vi "Convert RGB 1D Array to U32.vi"(9 "height":i32, 10 "width":i32, 11 "image":u8[](array[numeric])) -> (3 "output array":u32[][](array[numeric]) format="%.0x")   [LabVIEW 2025]
panel:
  out "?":u64[](array[numeric]) format="%.0x"
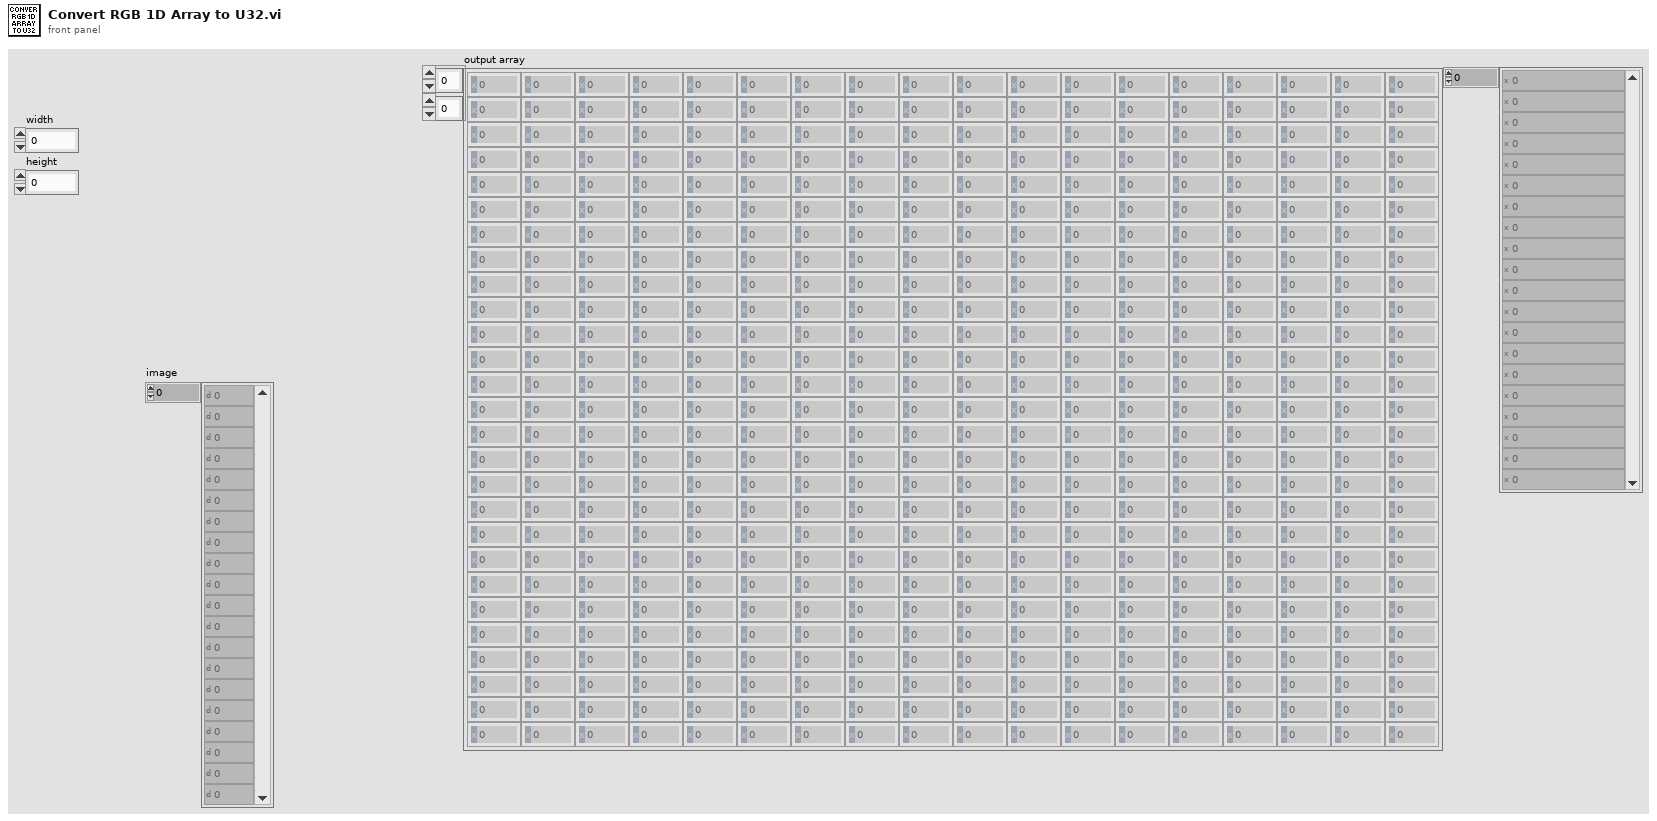
[diagram p1: front panel]
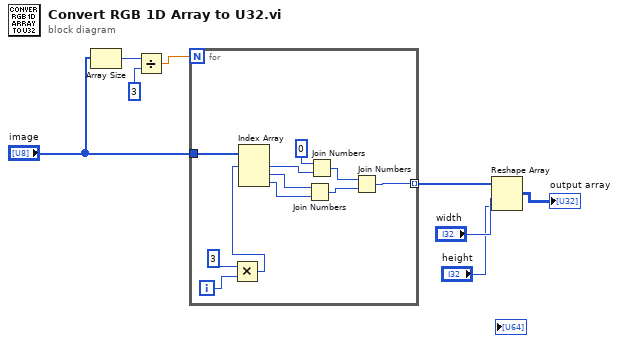
[diagram p0: block diagram]
diagram:
  n1 = Array Size(array="image") -> (size(s)=w4:i32)
  n2 = Divide(x=w4, y=3) -> (x/y=w1:dbl)
  n3 = for {
    N: w1 -> [_]
    tunnel: "image" -> [w16]
    tunnel: [w15] -> w8 mode=indexing
    i -> [w19]
    n4 = Multiply(x=3, y=w19) -> (x*y=w17:i32)
    n5 = Index Array(array=w16, index #1=w17) -> (element #1=w11:u8, element #2=w10:u8, element #3=w9:u8)  [unwired: 2 in]
    n6 = Join Numbers(hi=w10, lo=w9) -> ((hi.lo)=w12:u16)
    n7 = Join Numbers(hi=u8 0, lo=w11) -> ((hi.lo)=w13:u16)
    n8 = Join Numbers(hi=w13, lo=w12) -> ((hi.lo)=w15:u32)
  }
  n9 = Reshape Array(w8, "width", "height") -> (→"output array":u32[][])
